vi "split object path to hierarchy.vi"(11 "Object path":string="IndivITX/Test1/SA03008N.20190801.000000.itx") -> (1 "parent path":string, 2 "layers":i32, 3 "hierarchy":string[](array[string]))   [LabVIEW 2020, in "Data.S3.lvclass"]
uses:
  Data.S3.lvclass
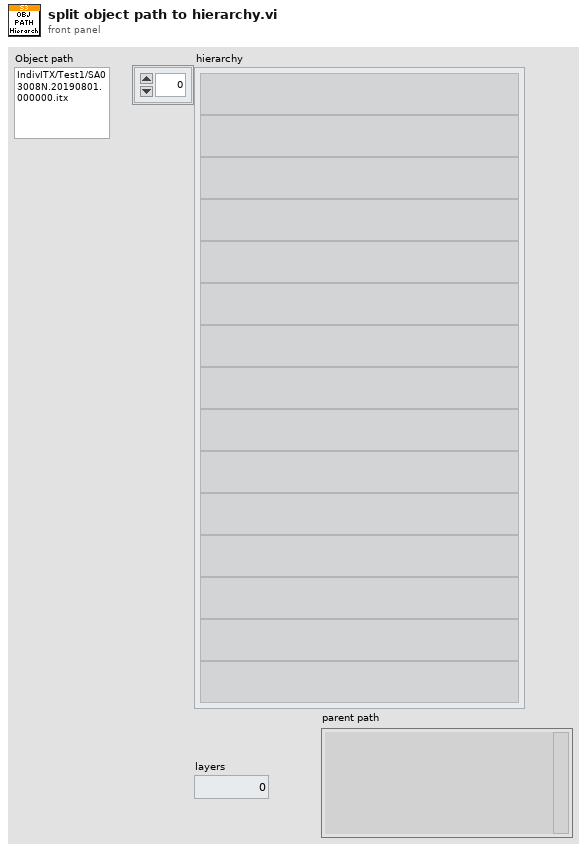
[diagram p1: front panel]
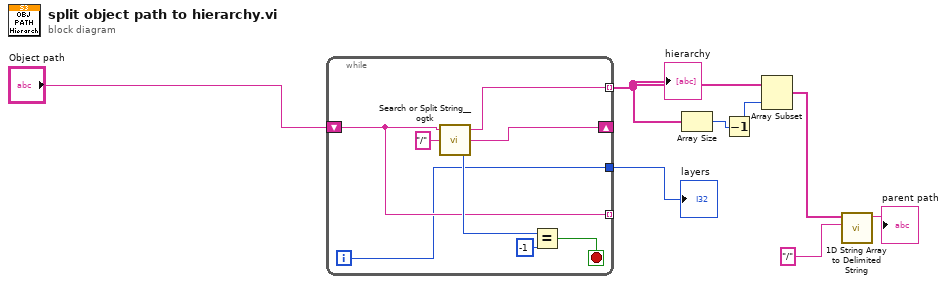
[diagram p0: block diagram]
diagram:
  n1 = while {
    shift-right: [w11] -> _
    shift-left: "Object path" -> [w12]
    tunnel: [w12] -> _ mode=indexing
    tunnel: [w10] -> w7
    tunnel: [w9] -> w6 mode=indexing
    i -> [w10]
    stop <- w13 stop-if-true
    n2 = call <userlib>:"Search or Split String__ogtk.vi"("search string/char (-)"="/", "string"=w12) -> ("offset after match"=w15:i32, "substring after match"=w11:string, "substring before match"=w9:string)  [unwired: 1 in]
    n3 = Equal?(x=w15, y=-1) -> (x = y?=w13:bool)
  }
  "hierarchy" <- w6
  "layers" <- w7
  n4 = Array Size(array=w6) -> (size(s)=w5:i32)
  n5 = Decrement(x=w5) -> (x-1=w4:i32)
  n6 = Array Subset(array=w6, length=w4) -> (w3:string[])  [unwired: 1 in]
  n7 = call <vilib>:"1D String Array to Delimited String.vi"("delimiter"="/", "string array"=w3) -> ("delimited string"=→"parent path":string)  [unwired: 9 in]
